vi "firstChildNodeData.vi"(8 "error in (no error)":errorcluster caption="errorIn", 11 "parentNode":refnum<k20>) -> (0 "error out":errorcluster caption="errorOut", 1 "data":string, 2 "childNode":refnum<k20>, 3 "parentNode":refnum<k20>)   [LabVIEW 2017]
uses:
  <vilib>/xml/NI_XML.lvlib
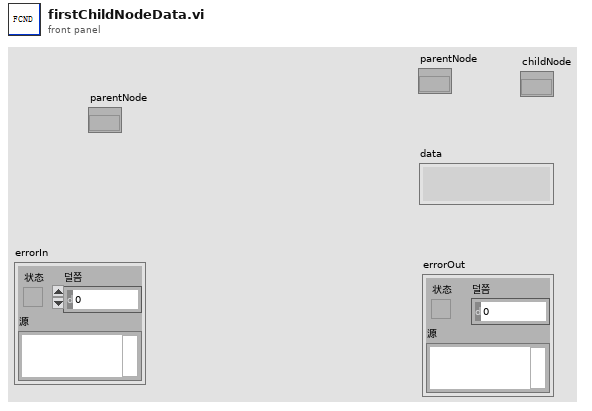
[diagram p1: front panel]
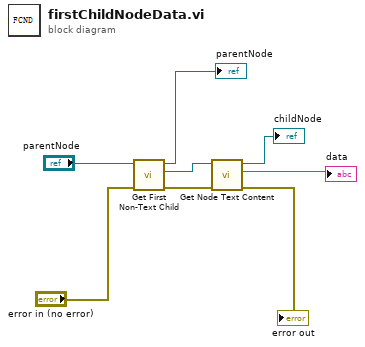
[diagram p0: block diagram]
diagram:
  n1 = call <vilib>:"Get First Non-Text Child.vi"("error in (no error)"="error in (no error)", "node in"="parentNode") -> ("error out"=w8:errorcluster, "child node"=w7:refnum<k20>, "node out"=→"parentNode":refnum<k20>)  [unwired: 7 out]
  n2 = call <vilib>:"Get Node Text Content.vi"("error in (no error)"=w8, "node in"=w7) -> ("error out"=→"error out":errorcluster, "node text"=→"data":string, "node out"=→"childNode":refnum<k20>)  [unwired: 7 out]
